vi "Amplitude cluster to array data.vi"(8 "Error In":errorcluster, 10 "Amplitude data":T1 {"Channel 31" min=0 max=204.8 step=0.0125 format="%#_g V"; "Channel 30" min=0 max=204.8 step=0.0125 format="%#_g V"; "Channel 29" min=0 max=204.8 step=0.0125 format="%#_g V"; "Channel 28" min=0 max=204.8 step=0.0125 format="%#_g V"; "Channel 27" min=0 max=204.8 step=0.0125 format="%#_g V"; "Channel 26" min=0 max=204.8 step=0.0125 format="%#_g V"; "Channel 25" min=0 max=204.8 step=0.0125 format="%#_g V"; "Channel 24" min=0 max=204.8 step=0.0125 format="%#_g V"; "Channel 23" min=0 max=204.8 step=0.0125 format="%#_g V"; "Channel 22" min=0 max=204.8 step=0.0125 format="%#_g V"; "Channel 21" min=0 max=204.8 step=0.0125 format="%#_g V"; "Channel 20" min=0 max=204.8 step=0.0125 format="%#_g V"; "Channel 19" min=0 max=204.8 step=0.0125 format="%#_g V"; "Channel 18" min=0 max=204.8 step=0.0125 format="%#_g V"; "Channel 17" min=0 max=204.8 step=0.0125 format="%#_g V"; "Channel 16" min=0 max=204.8 step=0.0125 format="%#_g V"; "Channel 15" min=0 max=204.8 step=0.0125 format="%#_g V"; "Channel 14" min=0 max=204.8 step=0.0125 format="%#_g V"; "Channel 13" min=0 max=204.8 step=0.0125 format="%#_g V"; "Channel 12" min=0 max=204.8 step=0.0125 format="%#_g V"; "Channel 11" min=0 max=204.8 step=0.0125 format="%#_g V"; "Channel 10" min=0 max=204.8 step=0.0125 format="%#_g V"; "Channel 9" min=0 max=204.8 step=0.0125 format="%#_g V"; "Channel 8" min=0 max=204.8 step=0.0125 format="%#_g V"; "Channel 7" min=0 max=204.8 step=0.0125 format="%#_g V"; "Channel 6" min=0 max=204.8 step=0.0125 format="%#_g V"; "Channel 5" min=0 max=204.8 step=0.0125 format="%#_g V"; "Channel 4" min=0 max=204.8 step=0.0125 format="%#_g V"; "Channel 3" min=0 max=204.8 step=0.0125 format="%#_g V"; "Channel 2" min=0 max=204.8 step=0.0125 format="%#_g V"; "Channel 1" min=0 max=204.8 step=0.0125 format="%#_g V"}) -> (0 "Error Out":errorcluster, 2 "Array data":dbl[](array[numeric]))   [LabVIEW 2016]
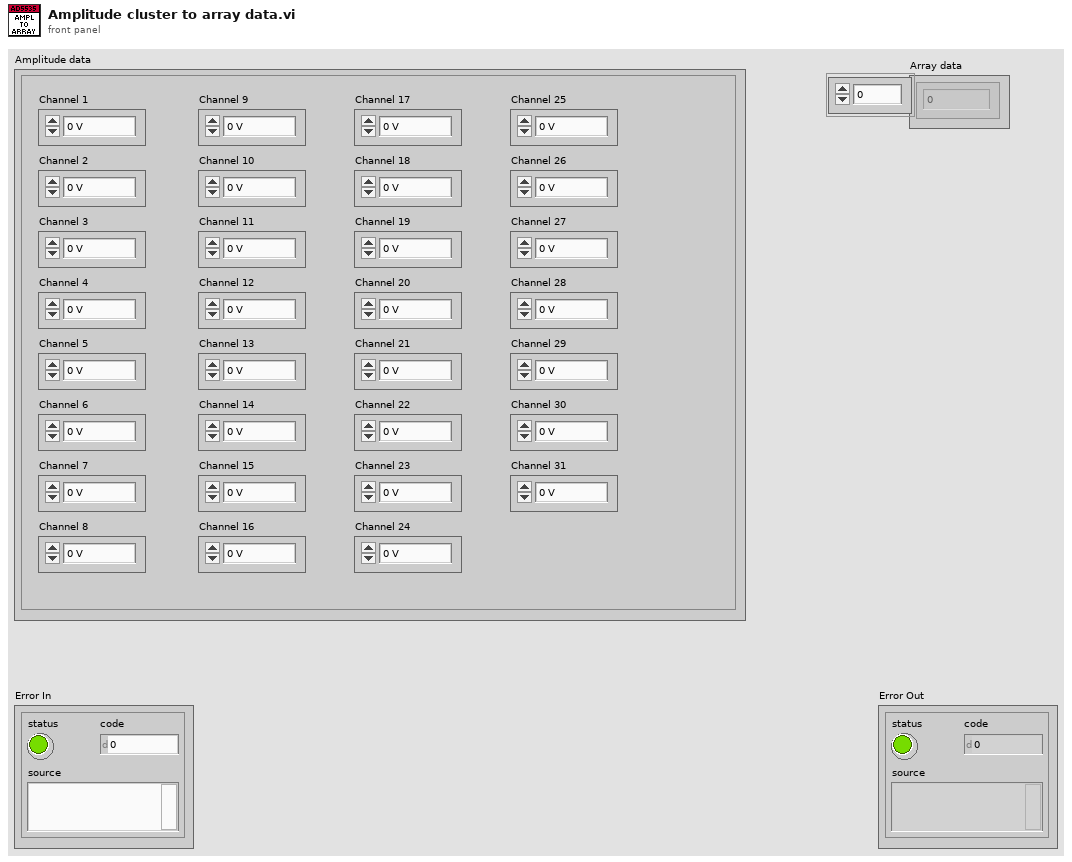
[diagram p1: front panel]
types:
  T1 = cluster{"Channel 1":sgl, "Channel 2":sgl, "Channel 3":sgl, "Channel 4":sgl, "Channel 5":sgl, "Channel 6":sgl, "Channel 7":sgl, "Channel 8":sgl, "Channel 9":sgl, "Channel 10":sgl, "Channel 11":sgl, "Channel 12":sgl, "Channel 13":sgl, "Channel 14":sgl, "Channel 15":sgl, "Channel 16":sgl, "Channel 17":sgl, "Channel 18":sgl, "Channel 19":sgl, "Channel 20":sgl, "Channel 21":sgl, "Channel 22":sgl, "Channel 23":sgl, "Channel 24":sgl, "Channel 25":sgl, "Channel 26":sgl, "Channel 27":sgl, "Channel 28":sgl, "Channel 29":sgl, "Channel 30":sgl, "Channel 31":sgl}
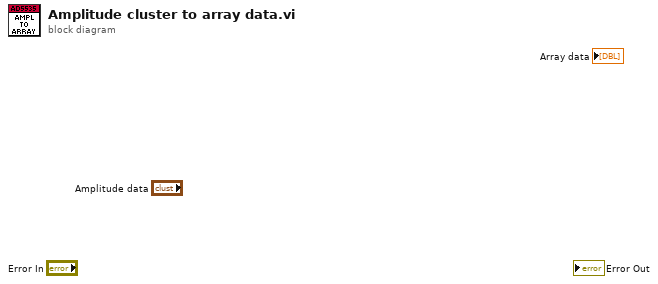
[diagram p0: block diagram]
diagram:
